vi "Кластеры-04-кластерошибок.vi"() -> ()   [LabVIEW 2017]
panel:
  out "Numeric 2":dbl
  in  "Numeric":dbl
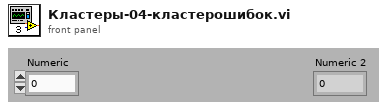
[diagram p1: front panel]
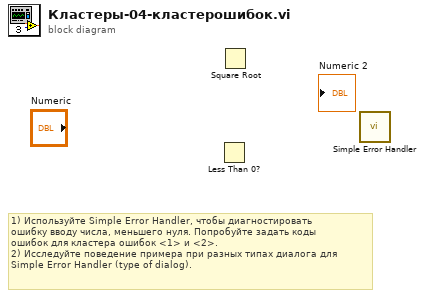
[diagram p0: block diagram]
diagram:
  # "1) Используйте Simple Error Handler, чтобы диагностировать \nошибку вводу числа, меньшего нуля. Попробуйте задать коды\nошибок для кластера ошибок <1> и <2>.\n2) Исследуйте поведение примера при разных типах диалога для\nSimple Error Handler (type of dialog)."
  n1 = Less Than 0?() -> ()  [unwired: 1 in, 1 out]
  n2 = Square Root() -> ()  [unwired: 1 in, 1 out]
  n3 = call <vilib>:"Simple Error Handler.vi"() -> ()  [unwired: 5 in, 5 out]
